vi "threshholdBestimmung.vi"() -> ()   [LabVIEW 2019]
panel:
  in  "File Name+Path":string
  out "Mid Count":u32
  out "Koinc Count":u32
  out "Bottom count":u32
  out "Or Count":u32
  out "Threshhold":i32
  in  "Wait time":u32
  in  "Start":i32
  in  "Step":i32
  out "Index":i32
  in  "Max Index":i32=16
  out "NemBox ID 2":string
  out "Versoion 2":string
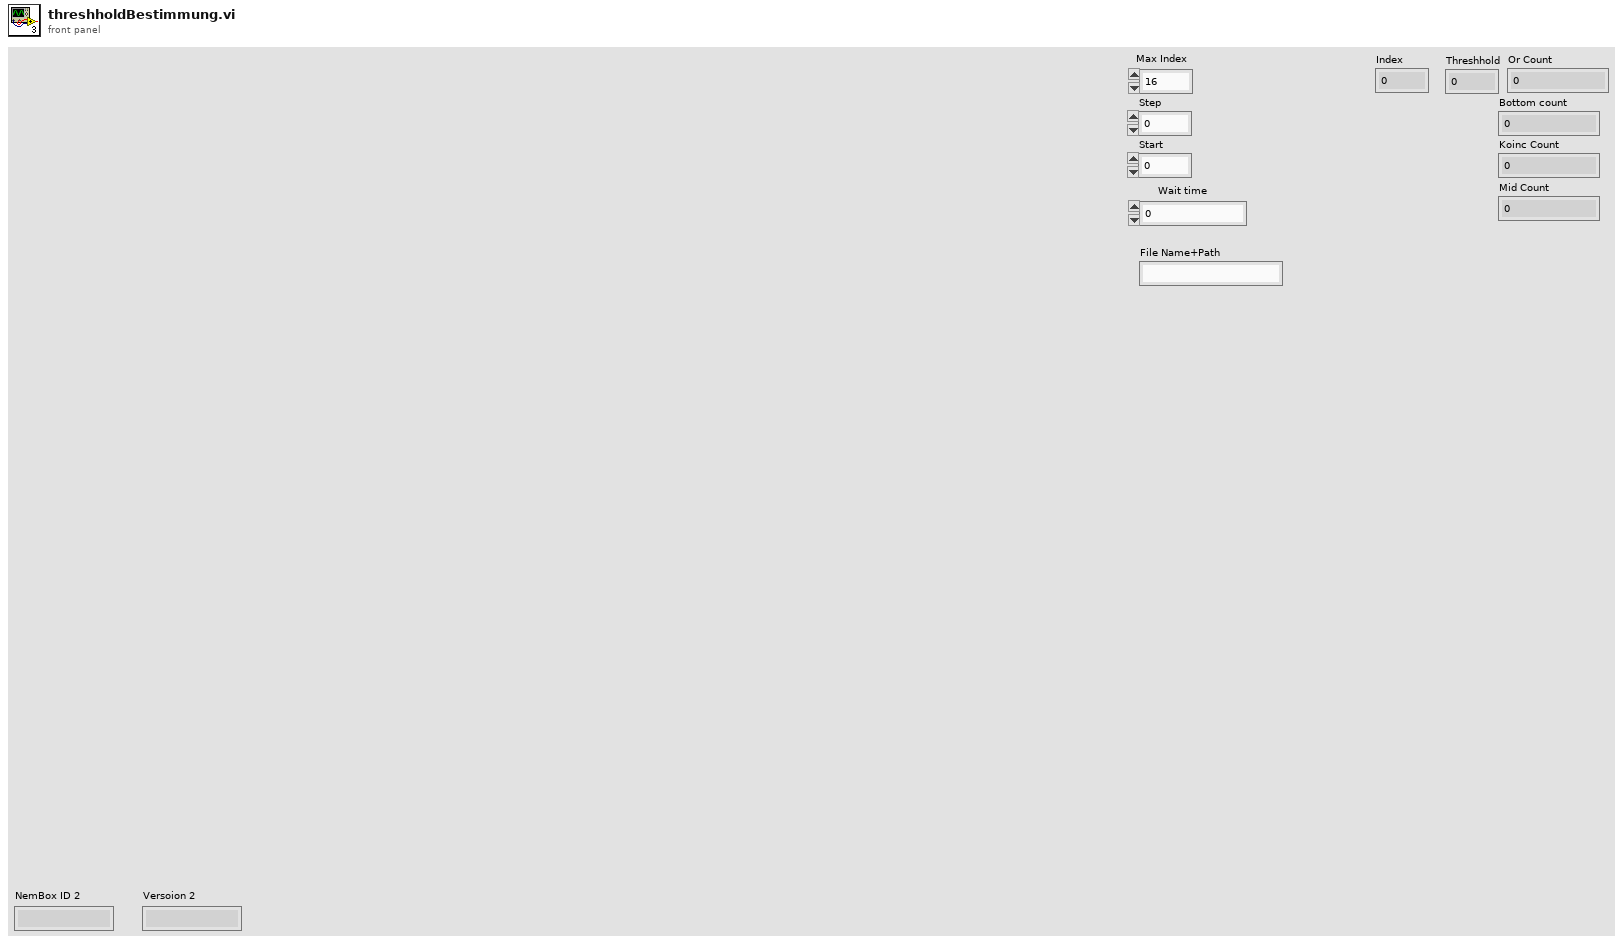
[diagram p1: front panel]
types:
  T1 = enum16{"Connect", "Set A", "Set B", "Set C", "Set D", "Set E", "Set F", "Set G", "Set H", "Get AND", "Read Counter", "Clear Counter"}
  T2 = enum16{"Connect", "Get IN", "Write Threshold", "Write Hysteresis", "Write Stretch"}
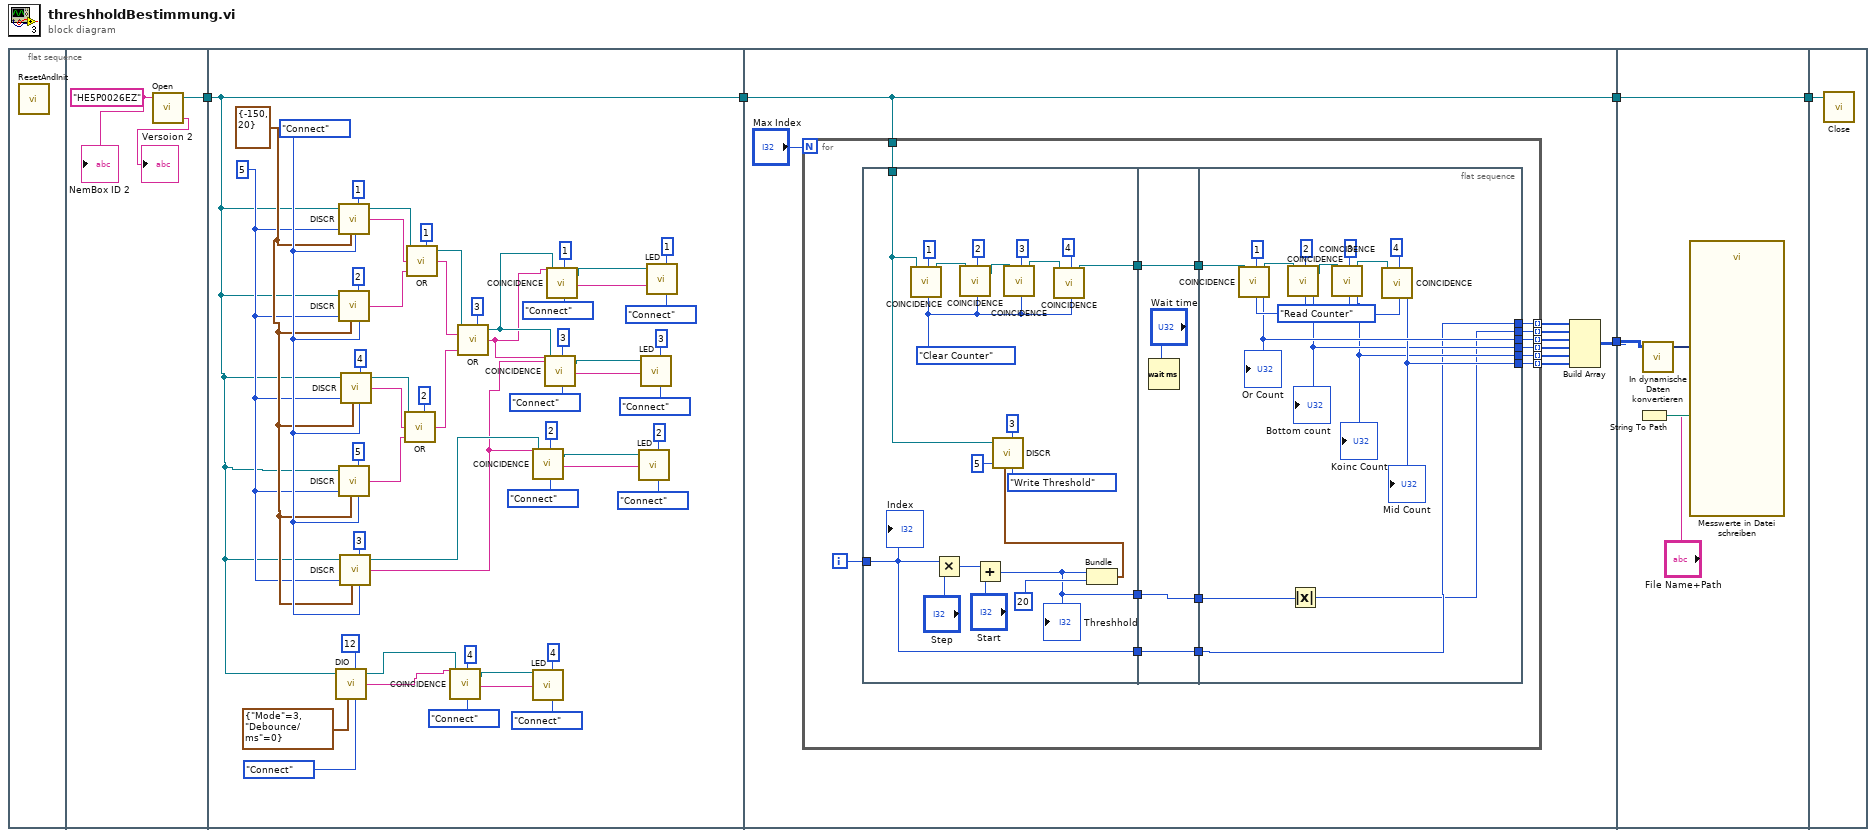
[diagram p0: block diagram]
diagram:
  n1 = flat-sequence {
    tunnel: [w8] -> w5
    tunnel: w5 -> [w40]
    tunnel: [w40] -> w4
    tunnel: [w71] -> w3
    tunnel: w4 -> [w71]
    tunnel: [w70] -> w1
    tunnel: w3 -> [w130]
    tunnel: [w130] -> w2
    tunnel: w1 -> [w127]
    tunnel: w2 -> [w131]
    frame #0 {
      n2 = call <userlib>:"ResetAndInit.vi"() -> ()  [unwired: 1 out]
    }
    frame #1 {
      w7 = "HE5P0026EZ"
      n3 = call <userlib>:"Open.vi"("USB_LogicBox"=w7) -> ("USB Out"=w8:refnum<visa-resource-name>, "Version"=→"Versoion 2":string)  [unwired: 1 in, 6 out]
      "NemBox ID 2" <- w7
    }
    frame #2 {
      w55 = u8 5 ("Stretch/10ns")
      w57 = T2."Connect" ("Function")
      w56 = cluster{"Threshold/mV":i16, "Hysteresis/mV":u16} {"Threshold/mV"=-150, "Hysteresis/mV"=20} ("Params")
      n4 = call <userlib>:"DIO.vi"("USB In"=w40, "Params"=cluster{"Mode":u8, "Debounce/ms":u8} {"Mode"=3, "Debounce/ms"=0}, "DIO#"=u8 12, "Function"=enum16{"Connect", "Set DO", "Get DI"}."Connect") -> ("USB Out"=w38:refnum<visa-resource-name>, "DI"=w37:string)  [unwired: 1 in, 3 out]
      n5 = call <userlib>:"DISCR.vi"("USB In"=w40, "Stretch/10ns"=w55, "Params"=w56, "DISCR#"=u8 1, "Function"=w57) -> ("USB Out"=w54:refnum<visa-resource-name>, "DISCR"=w53:string)  [unwired: 3 in]
      n6 = call <userlib>:"DISCR.vi"("USB In"=w40, "Stretch/10ns"=w55, "Params"=w56, "DISCR#"=u8 2, "Function"=w57) -> ("DISCR"=w52:string)  [unwired: 3 in, 1 out]
      n7 = call <userlib>:"DISCR.vi"("USB In"=w40, "Stretch/10ns"=w55, "Params"=w56, "DISCR#"=u8 5, "Function"=w57) -> ("DISCR"=w49:string)  [unwired: 3 in, 1 out]
      n8 = call <userlib>:"DISCR.vi"("USB In"=w40, "Stretch/10ns"=w55, "Params"=w56, "DISCR#"=u8 3, "Function"=w57) -> ("USB Out"=w28:refnum<visa-resource-name>, "DISCR"=w27:string)  [unwired: 3 in]
      n9 = call <userlib>:"DISCR.vi"("USB In"=w40, "Stretch/10ns"=w55, "Params"=w56, "DISCR#"=u8 4, "Function"=w57) -> ("USB Out"=w51:refnum<visa-resource-name>, "DISCR"=w50:string)  [unwired: 3 in]
      n10 = call <userlib>:"OR.vi"("USB In"=w51, "A"=w50, "B"=w49, "LOGIC#"=u8 2) -> ("OR"=w45:string)  [unwired: 1 in, 4 out]
      n11 = call <userlib>:"OR.vi"("USB In"=w54, "A"=w53, "B"=w52, "LOGIC#"=u8 1) -> ("USB Out"=w44:refnum<visa-resource-name>, "OR"=w46:string)  [unwired: 1 in, 3 out]
      n12 = call <userlib>:"COINCIDENCE.vi"("A"=w37, "USB In"=w38, "CC#"=u8 4, "Function"=T1."Connect") -> ("USB Out"=w34:refnum<visa-resource-name>, "AND"=w33:string)  [unwired: 21 in, 1 out]
      n13 = call <userlib>:"OR.vi"("USB In"=w44, "A"=w46, "B"=w45, "LOGIC#"=u8 3) -> ("USB Out"=w30:refnum<visa-resource-name>, "OR"=w29:string)  [unwired: 1 in, 3 out]
      n14 = call <userlib>:"COINCIDENCE.vi"("A"=w27, "USB In"=w28, "CC#"=u8 2, "Function"=T1."Connect") -> ("USB Out"=w13:refnum<visa-resource-name>, "AND"=w12:string)  [unwired: 21 in, 1 out]
      n15 = call <userlib>:"LED.vi"("USB In"=w34, "STATE"=w33, "LED#"=u8 4, "Function"=enum16{"Connect", "Set STATE"}."Connect") -> ()  [unwired: 5 in, 1 out]
      n16 = call <userlib>:"COINCIDENCE.vi"("A"=w29, "B"=w27, "USB In"=w30, "CC#"=u8 3, "Function"=T1."Connect") -> ("USB Out"=w15:refnum<visa-resource-name>, "AND"=w14:string)  [unwired: 20 in, 1 out]
      n17 = call <userlib>:"COINCIDENCE.vi"("A"=w29, "USB In"=w30, "CC#"=u8 1, "Function"=T1."Connect") -> ("USB Out"=w17:refnum<visa-resource-name>, "AND"=w16:string)  [unwired: 21 in, 1 out]
      n18 = call <userlib>:"LED.vi"("USB In"=w13, "STATE"=w12, "LED#"=u8 2, "Function"=enum16{"Connect", "Set STATE"}."Connect") -> ()  [unwired: 5 in, 1 out]
      n19 = call <userlib>:"LED.vi"("USB In"=w15, "STATE"=w14, "LED#"=u8 3, "Function"=enum16{"Connect", "Set STATE"}."Connect") -> ()  [unwired: 5 in, 1 out]
      n20 = call <userlib>:"LED.vi"("USB In"=w17, "STATE"=w16, "LED#"=u8 1, "Function"=enum16{"Connect", "Set STATE"}."Connect") -> ()  [unwired: 5 in, 1 out]
    }
    frame #3 {
      n21 = for {
        N: "Max Index" -> [_]
        tunnel: w71 -> [w84]
        tunnel: [w77] -> w69 mode=indexing
        tunnel: [w76] -> w68 mode=indexing
        tunnel: [w75] -> w67 mode=indexing
        tunnel: [w74] -> w66 mode=indexing
        tunnel: [w73] -> w65 mode=indexing
        tunnel: [w72] -> w64 mode=indexing
        i -> [w85]
        n22 = flat-sequence {
          tunnel: w85 -> [w86]
          tunnel: w84 -> [w94]
          tunnel: [w89] -> w82
          tunnel: [w87] -> w81
          tunnel: [w86] -> w79
          tunnel: [w108] -> w83
          tunnel: w82 -> [w108]
          tunnel: w81 -> [w107]
          tunnel: [w107] -> w80
          tunnel: w79 -> [w106]
          tunnel: [w106] -> w78
          tunnel: w83 -> [w117]
          tunnel: w80 -> [w110]
          tunnel: w78 -> [w112]
          tunnel: [w116] -> w77
          tunnel: [w114] -> w76
          tunnel: [w113] -> w75
          tunnel: [w115] -> w74
          tunnel: [w112] -> w73
          tunnel: [w111] -> w72
          frame #0 {
            w90 = T1."Clear Counter" ("Function")
            n23 = call <userlib>:"COINCIDENCE.vi"("USB In"=w94, "CC#"=u8 1, "Function"=w90) -> ("USB Out"=w93:refnum<visa-resource-name>)  [unwired: 22 in, 2 out]
            n24 = Multiply(x=w86, y="Step") -> (x*y=w104:i32)
            n25 = call <userlib>:"COINCIDENCE.vi"("USB In"=w93, "CC#"=u8 2, "Function"=w90) -> ("USB Out"=w92:refnum<visa-resource-name>)  [unwired: 22 in, 2 out]
            n26 = Add(x=w104, y="Start") -> (x+y=w87:i32)
            "Threshhold" <- w87
            n27 = call <userlib>:"COINCIDENCE.vi"("USB In"=w92, "CC#"=u8 3, "Function"=w90) -> ("USB Out"=w91:refnum<visa-resource-name>)  [unwired: 22 in, 2 out]
            n28 = call <userlib>:"COINCIDENCE.vi"("USB In"=w91, "CC#"=u8 4, "Function"=w90) -> ("USB Out"=w89:refnum<visa-resource-name>)  [unwired: 22 in, 2 out]
            n29 = Bundle(w87, "Hysteresis/mV"=u16 20) -> (w88:cluster{i32, "Hysteresis/mV":u16})  [unwired: 1 out]
            n30 = call <userlib>:"DISCR.vi"("USB In"=w94, "Stretch/10ns"=u8 5, "Params"=w88, "DISCR#"=u8 3, "Function"=T2."Write Threshold") -> ()  [unwired: 3 in, 2 out]
            "Index" <- w86
          }
          frame #1 {
            n31 = Wait (ms)(milliseconds to wait="Wait time") -> ()  [unwired: 1 out]
          }
          frame #2 {
            w118 = T1."Read Counter" ("Function")
            n32 = call <userlib>:"COINCIDENCE.vi"("USB In"=w117, "CC#"=u8 1, "Function"=w118) -> ("USB Out"=w121:refnum<visa-resource-name>, "Counter"=w116:u32)  [unwired: 22 in, 1 out]
            "Or Count" <- w116
            n33 = call <userlib>:"COINCIDENCE.vi"("USB In"=w121, "CC#"=u8 2, "Function"=w118) -> ("USB Out"=w120:refnum<visa-resource-name>, "Counter"=w114:u32)  [unwired: 22 in, 1 out]
            "Bottom count" <- w114
            n34 = Absolute Value(x=w110) -> (abs(x)=w111:i32)
            n35 = call <userlib>:"COINCIDENCE.vi"("USB In"=w120, "CC#"=u8 3, "Function"=w118) -> ("USB Out"=w119:refnum<visa-resource-name>, "Counter"=w113:u32)  [unwired: 22 in, 1 out]
            "Koinc Count" <- w113
            n36 = call <userlib>:"COINCIDENCE.vi"("USB In"=w119, "CC#"=u8 4, "Function"=w118) -> ("Counter"=w115:u32)  [unwired: 22 in, 2 out]
            "Mid Count" <- w115
          }
        }
      }
      n37 = Build Array(w65, w64, w69, w68, w67, w66) -> (w70:u32[][])
    }
    frame #4 {
      n38 = String To Path(string="File Name+Path") -> (path=w129:path)
      n39 = call "In dynamische Daten konvertieren"("2D Array"=w127) -> ("Dynamic Data Type"=w128:dynamicdata)  [unwired: 3 out]
      n40 = call "Messwerte in Datei schreiben"("Signals"=w128, "Filename"=w129) -> ()  [unwired: 15 in, 3 out]
    }
    frame #5 {
      n41 = call <userlib>:"Close.vi"("USB In"=w131) -> ()  [unwired: 1 in, 8 out]
    }
  }
